vi "myRIOXC Validate Data.vi"(9 "Size":i32, 11 "Data In":bool[](array[boolean])) -> (1 "Data Changed?":bool, 3 "Data Out":bool[](array[boolean]))   [LabVIEW 2021]
doc: "This VI validates the size of data is corresponding to \nconnector type."
panel:
  # "This VI validates the size of data is corresponding to \nconnector type."
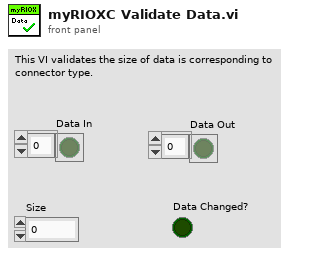
[diagram p1: front panel]
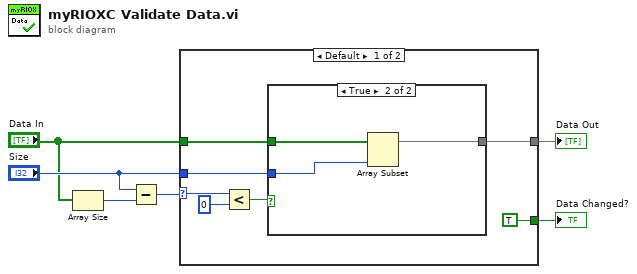
[diagram p0: block diagram]
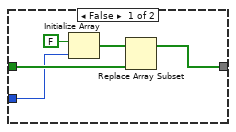
[diagram p2: hidden frame]
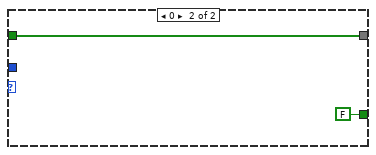
[diagram p3: hidden frame]
diagram:
  n1 = Array Size(array="Data In") -> (size(s)=w6:i32)
  n2 = Subtract(x="Size", y=w6) -> (x-y=w5:i32)
  n3 = case shown="Default" w5 {
    selector: w5 -> [w13 _]
    tunnel: "Data In" -> [w9 w23]
    tunnel: [w8 w23] -> w4
    tunnel: "Size" -> [w10 _]
    tunnel: [TRUE ("Data Changed?") FALSE ("Data Changed?")] -> w1
    frame Default {
      n4 = Less?(x=w13, y=0) -> (x < y?=w11:bool)
      n5 = case shown="True" w11 {
        tunnel: w10 -> [w14 w20]
        tunnel: w9 -> [w16 w21]
        tunnel: [w15 w19] -> w8
        frame False {
          n6 = Initialize Array(FALSE, w14) -> (w17:bool[])
          n7 = Replace Array Subset(array=w17, new element=w16) -> (w15:bool[])  [unwired: 1 in]
        }
        frame True {
          n8 = Array Subset(array=w21, length=w20) -> (w19:bool[])  [unwired: 1 in]
        }
      }
    }
    frame 0 {
    }
  }
  "Data Out" <- w4
  "Data Changed?" <- w1
